vi "SiosIfmI2CReadValue.vi"(1 "Index":i32, 2 "Device Number":i32) -> (0 "i2c Value":string)   [LabVIEW 2009]
uses:
  siosifm.dll
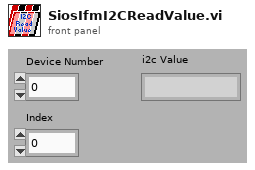
[diagram p1: front panel]
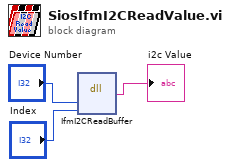
[diagram p0: block diagram]
diagram:
  n1 = dll-call lib="C:/WORK/Artem/RE-10/SIOS_IfmDLL/siosifm.dll" fn="IfmI2CReadBuffer"("devNumber"="Device Number", "Index"="Index") -> ("i2c Buffer"=→"i2c Value":string)  [unwired: 5 in, 2 out]
